vi "Get Subtype Description.vi"(8 "error in (no error)":errorcluster, 11 "Boolean Assertion in":refnum<class "Boolean Assertion.lvclass">) -> (0 "error out":errorcluster, 2 "Subtype Description":string, 3 "Boolean Assertion out":refnum<class "Boolean Assertion.lvclass">)   [LabVIEW 2020, in "MacroAssert.lvlib" / "Boolean Assertion.lvclass"]
doc: "Gets the subtype description for <B>Step in</B>, which describes what the step's subtype does specifically."
uses:
  Boolean Assertion.lvclass
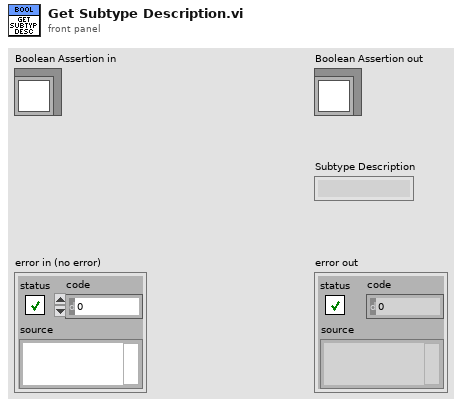
[diagram p1: front panel]
types:
  T1 = typedef "MacroAssert.lvlib/Boolean Assertion.lvclass/Boolean Assertion Type.ctl" = enum16{"Boolean Ctl Value", "Ctl Visible Property", "Ctl is Enabled", "Ctl is Grayed Out", "Ctl Key Focus Property", "VI Front Panel is Open", "Window is in Running Windows", "Window is in Monitor Bounds"}
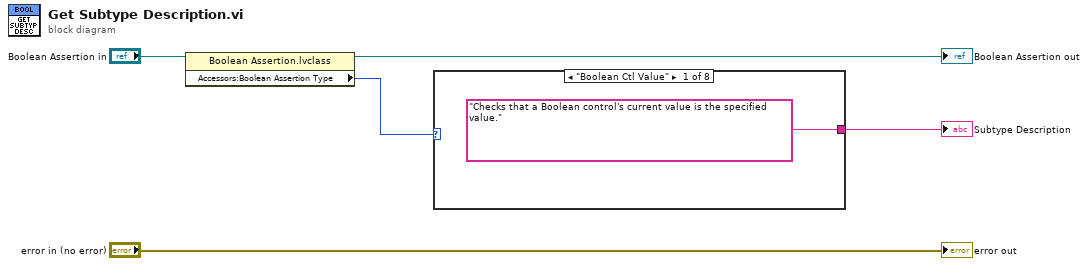
[diagram p0: block diagram]
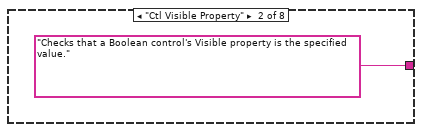
[diagram p2: hidden frame]
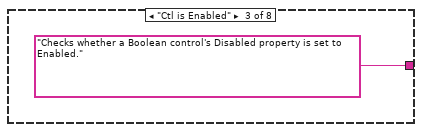
[diagram p3: hidden frame]
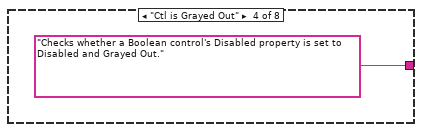
[diagram p4: hidden frame]
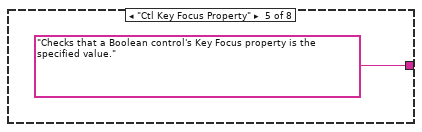
[diagram p5: hidden frame]
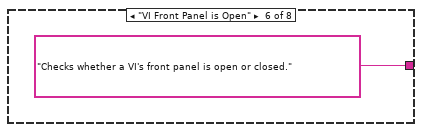
[diagram p6: hidden frame]
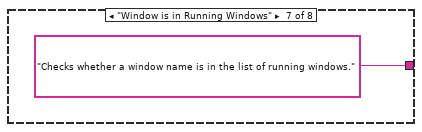
[diagram p7: hidden frame]
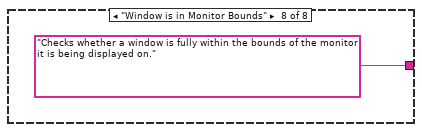
[diagram p8: hidden frame]
diagram:
  n1 = property class="Boolean Assertion.lvclass"(reference="Boolean Assertion in") -> (reference out=→"Boolean Assertion out":refnum<class "Boolean Assertion.lvclass">, "Accessors:Boolean Assertion Type"=w2:T1)  [unwired: 1 in, 1 out]
  n2 = case shown="\"Boolean Ctl Value\"" w2 {
    tunnel: ["Checks that a Boolean control's current value is the specified value." "Checks that a Boolean control's Visible property is the specified value." "Checks whether a Boolean control's Disabled property is set to Enabled." "Checks whether a Boolean control's Disabled property is set to Disabled and Grayed Out." "Checks that a Boolean control's Key Focus property is the specified value." "Checks whether a VI's front panel is open or closed." "Checks whether a window name is in the list of running windows." "Checks whether a window is fully within the bounds of the monitor it is being displayed on."] -> w1
    frame "Boolean Ctl Value" {
    }
    frame "Ctl Visible Property" {
    }
    frame "Ctl is Enabled" {
    }
    frame "Ctl is Grayed Out" {
    }
    frame "Ctl Key Focus Property" {
    }
    frame "VI Front Panel is Open" {
    }
    frame "Window is in Running Windows" {
    }
    frame "Window is in Monitor Bounds" {
    }
  }
  "Subtype Description" <- w1
  "error out" <- "error in (no error)"
